vi "Open.vi"(8 "Error In":errorcluster, 9 "CS Channel":u8, 10 "SPI Channel (0)":u8, 11 "LINX Resource":T1) -> (0 "Error Out":errorcluster, 3 "LINX Resource":T1)   [LabVIEW 2011, in "LVH-LINX.lvlib" / "AD9850.lvlib"]
uses:
  AD9850.lvlib
  Private/Type Defs/LINX Ref.ctl
  Private/Type Defs/Platform.ctl
  Private/Type Defs/Interface.ctl
  Private/Device/Type Defs/LINX Device Config.ctl
  Private/Device/Type Defs/TCP Config.ctl
  Private/Type Defs/Device Family.ctl
  Private/Type Defs/Peripherals/SPI/SPI Configuration.ctl
  Private/Type Defs/Peripherals/SPI/SPI Bit Order.ctl
  Private/Type Defs/Peripherals/SPI/SPI Clock Phase.ctl
  Private/Type Defs/Peripherals/SPI/SPI Clock Polarity.ctl
  Private/Type Defs/Peripherals/SPI/SPI CS Logic Level.ctl
  LVH-LINX.lvlib
  Private/Device/Device.lvlib
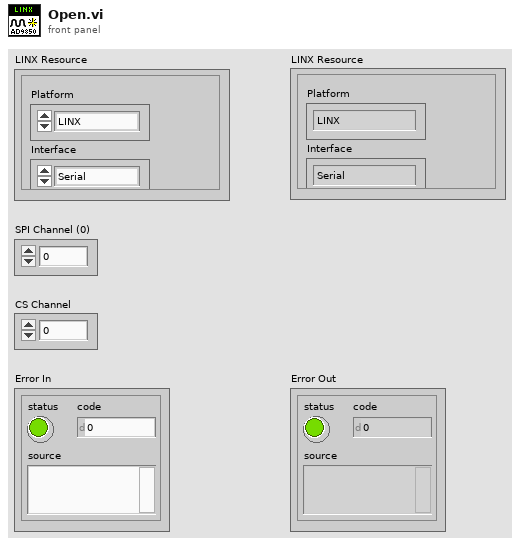
[diagram p1: front panel]
types:
  T1 = typedef "LVH-LINX.lvlib/LINX Ref.ctl" = cluster{"Platform":T2, "Interface":T3, "LINX Device Config":T4}
  T2 = typedef "LVH-LINX.lvlib/Platform.ctl" = enum16{"LINX", "myRIO"}
  T3 = typedef "LVH-LINX.lvlib/Interface.ctl" = enum16{"Serial", "TCP"}
  T4 = typedef "LVH-LINX.lvlib/Device.lvlib/LINX Device Config.ctl" = cluster{"Interface":T3, "COM Port":refnum<visa-resource-name>, "TCP Configuration":T5, "Device Family":T6, "Device ID":u8, "Device Name":string, "TCP Ref":refnum<k5>}
  T5 = typedef "LVH-LINX.lvlib/Device.lvlib/TCP Config.ctl" = cluster{"IP Address":string, "Port":u16}
  T6 = typedef "LVH-LINX.lvlib/Device Family.ctl" = enum8{"National Instruments", "Digilent", "Arduino"}
  T7 = typedef "LVH-LINX.lvlib/SPI Configuration.ctl" = cluster{"Clock Frequency":u32, "Bit Order":T8, "CLK Phase":T9, "CLK Polarity":T10, "Frame Size (Bytes)":u8, "CS Channel":u8, "CS Logic Level":T11}
  T8 = typedef "LVH-LINX.lvlib/SPI Bit Order.ctl" = enum8{"LSb First", "MSb First"}
  T9 = typedef "LVH-LINX.lvlib/SPI Clock Phase.ctl" = enum8{"Leading", "Trailing"}
  T10 = typedef "LVH-LINX.lvlib/SPI Clock Polarity.ctl" = enum8{"Idle Low", "Idle High"}
  T11 = typedef "LVH-LINX.lvlib/SPI CS Logic Level.ctl" = enum8{"Active Low", "Active High"}
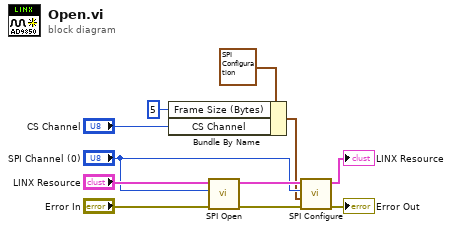
[diagram p0: block diagram]
diagram:
  n1 = Bundle By Name(cluster=T7 {"Clock Frequency"=0, "Bit Order"=enum."LSb First", "CLK Phase"=enum."Leading", "CLK Polarity"=enum."Idle Low", "Frame Size (Bytes)"=0, "CS Channel"=0, "CS Logic Level"=enum."Active Low"} ("SPI Configuration"), "Frame Size (Bytes)"=u8 5, "CS Channel"="CS Channel") -> (w3:T7)
  n2 = call "SPI Open.vi"("Error In"="Error In", "SPI Channel (0)"="SPI Channel (0)", "LINX Resource"="LINX Resource") -> ("Error Out"=w8:errorcluster, "LINX Resource"=w9:T1)  [unwired: 7 in]
  n3 = call "SPI Configure.vi"("Error In"=w8, "SPI Configuration"=w3, "SPI Channel (0)"="SPI Channel (0)", "LINX Resource"=w9) -> ("Error Out"=→"Error Out":errorcluster, "LINX Resource"=→"LINX Resource":T1)  [unwired: 6 in]
